vi "water flow.vi"(5 "Time":dbl format="%.2f", 6 "sensor value":dbl, 7 "Set Points":dbl[](array[numeric])) -> (3 "fraction on":dbl)   [LabVIEW 2010]
panel:
  out "valve state":enum16{"closed", "open"}(ring)
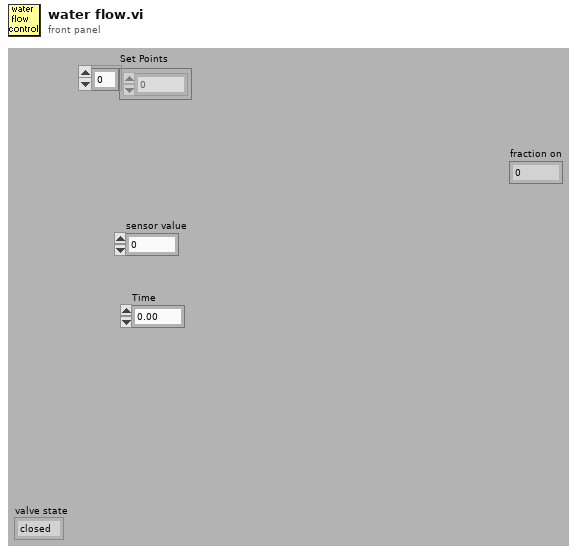
[diagram p1: front panel]
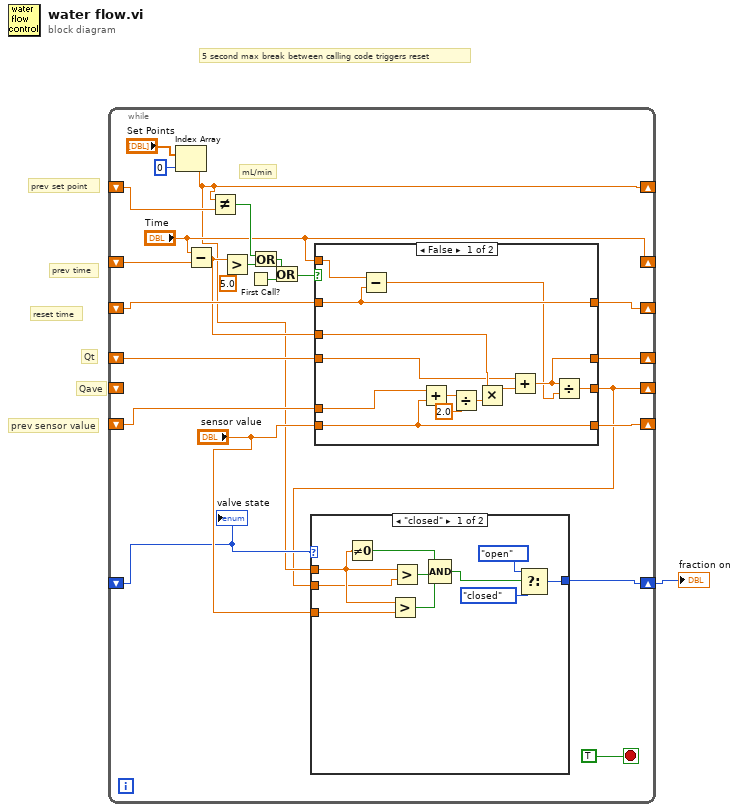
[diagram p0: block diagram]
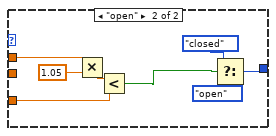
[diagram p2: hidden frame]
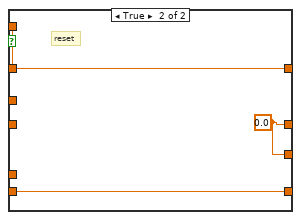
[diagram p3: hidden frame]
diagram:
  # "Qave"
  # "reset time"
  # "Qt"
  # "prev sensor value"
  # "5 second max break between calling code triggers reset"
  # "prev time"
  # "prev set point"
  n1 = while {
    shift-right: [w3] -> _
    shift-left: _ -> [w23]
    shift-right: ["Time"] -> _
    shift-left: _ -> [w22]
    shift-right: [w8] -> _
    shift-left: _ -> [w10]
    shift-right: [w12] -> _
    shift-left: _ -> [w9]
    shift-right: [w15] -> _
    shift-left: _ -> [w13]
    shift-right: [w2] -> _
    shift-left: _ -> [_]
    shift-right: [w5] -> w1
    shift-left: _ -> [w4]
    stop <- TRUE stop-if-true
    # "mL/min"
    n2 = Index Array(array="Set Points", index=0) -> (element=w3:dbl)
    n3 = Subtract(x="Time", y=w22) -> (x-y=w11:dbl)
    n4 = Not Equal?(x=w3, y=w23) -> (x != y?=w20:bool)
    n5 = Greater?(x=w11, y=5.0) -> (0:w19:bool)
    n6 = First Call?() -> (First Call?: T/F=w18:bool)
    n7 = Or(x=w20, y=w19) -> (x .or. y?=w17:bool)
    n8 = Or(x=w17, y=w18) -> (x .or. y?=w16:bool)
    n9 = case shown="False" w16 {
      tunnel: [w46 w59] -> w15
      tunnel: "Time" -> [w47 w59]
      tunnel: w13 -> [w46 _]
      tunnel: [w48 w57] -> w12
      tunnel: w11 -> [w52 _]
      tunnel: w10 -> [w51 _]
      tunnel: "sensor value" -> [w49 w58]
      tunnel: w9 -> [w50 _]
      tunnel: [w49 w58] -> w8
      tunnel: [w44 w57] -> w2
      frame False {
        n10 = Subtract(x=w47, y=w46) -> (x-y=w45:dbl)
        n11 = Add(x=w51, y=w49) -> (x+y=w53:dbl)
        n12 = Divide(x=w53, y=2.0) -> (x/y=w55:dbl)
        n13 = Multiply(x=w52, y=w55) -> (x*y=w56:dbl)
        n14 = Add(x=w50, y=w56) -> (x+y=w48:dbl)
        n15 = Divide(x=w48, y=w45) -> (x/y=w44:dbl)
      }
      frame True {
        w57 = 0.0 ("y")
        # "reset"
      }
    }
    n16 = case shown="\"closed\"" w4 {
      tunnel: [w35 w43] -> w5
      tunnel: w3 -> [w28 w42]
      tunnel: "sensor value" -> [w29 w39]
      tunnel: w2 -> [w26 _]
      frame "closed" {
        n17 = Not Equal To 0?(x=w28) -> (x != 0?=w32:bool)
        n18 = Greater?(x=w28, y=w29) -> (0:w27:bool)
        n19 = Greater?(x=w28, y=w26) -> (0:w34:bool)
        n20 = Compound Arithmetic op=AND(w32, w34, w27) -> (w33:bool)
        n21 = Select(t=enum16{"closed", "open"}."open" ("valve state"), s=w33, f=enum16{"closed", "open"}."closed" ("valve state")) -> (s? t:f=w35:enum16{"closed", "open"})
      }
      frame "open" {
        n22 = Multiply(x=w42, y=1.05) -> (x*y=w41:dbl)
        n23 = Less?(x=w41, y=w39) -> (x < y?=w36:bool)
        n24 = Select(t=enum16{"closed", "open"}."closed" ("valve state"), s=w36, f=enum16{"closed", "open"}."open" ("valve state")) -> (s? t:f=w43:enum16{"closed", "open"})
      }
    }
    "valve state" <- w4
  }
  "fraction on" <- w1
